vi "SetDirection.vi"(8 "error in (no error)":errorcluster, 10 "Direction":csg, 11 "reference in":refnum<class "Sprite.lvclass">) -> (0 "error out":errorcluster, 3 "reference out":refnum<class "Sprite.lvclass">)   [LabVIEW 2010, in "RenderBase.lvlib" / "Sprite.lvclass"]
uses:
  Sprite.lvclass
  Sprite.lvclass/Sprite.ctl
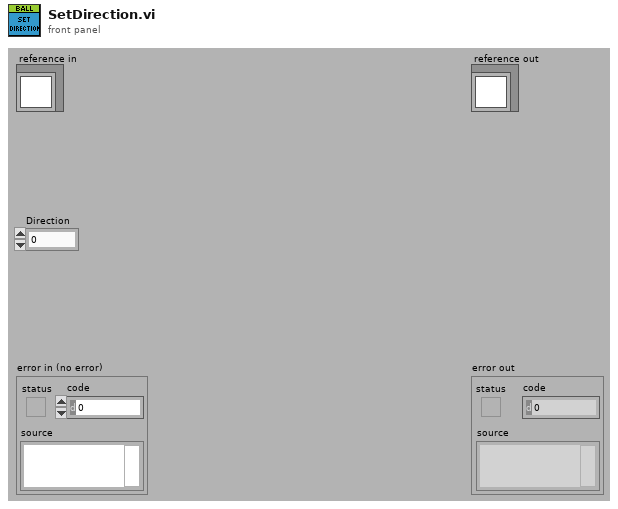
[diagram p1: front panel]
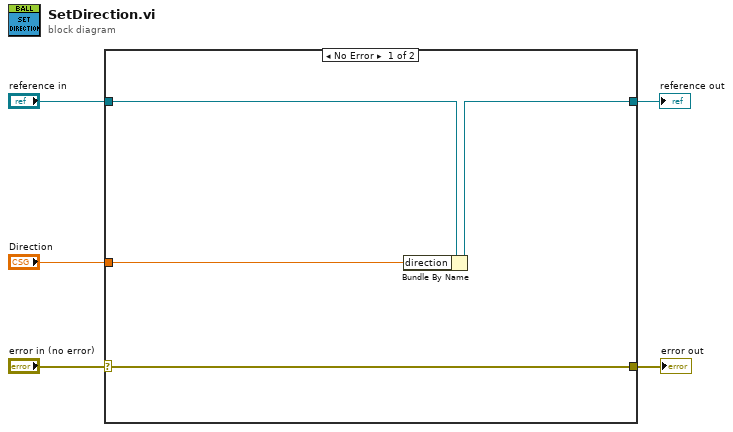
[diagram p0: block diagram]
diagram:
  n1 = case shown="No Error" "error in (no error)" {
    selector: "error in (no error)" -> [w6 w11]
    tunnel: [w6 w11] -> w4
    tunnel: [w8 w10] -> w2
    tunnel: "reference in" -> [w9 w10]
    tunnel: "Direction" -> [w7 _]
    frame No Error {
      n2 = Bundle By Name(cluster=w9, "direction"=w7) -> (w8:refnum<class "Sprite.lvclass">)
    }
    frame Error {
    }
  }
  "error out" <- w4
  "reference out" <- w2
